vi "Address Lookup Table Initialize.vi"(8 "error in (no error)":errorcluster) -> (0 "error out":errorcluster {"code" min=0 max=0}, 3 "reference out 2":T1)   [LabVIEW 2013, in "J1939 Addon Engine.lvlib"]
uses:
  J1939 Addon Engine.lvlib
  Shared/J1939 Multi Packet Frame/Types/Address Table Reference.ctl
  Shared/J1939 Multi Packet Frame/Types/Address Lookup Table Action.ctl
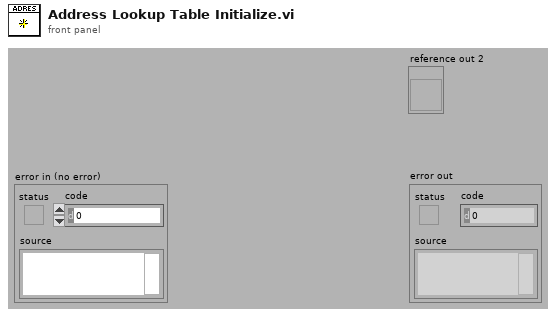
[diagram p1: front panel]
types:
  T1 = typedef "J1939 Addon Engine.lvlib/Address Table Reference.ctl" = refnum<vi>
  T2 = typedef "J1939 Addon Engine.lvlib/Address Lookup Table Action.ctl" = enum16{"Initialize", "Add", "Get", "Remove", "Get All"}
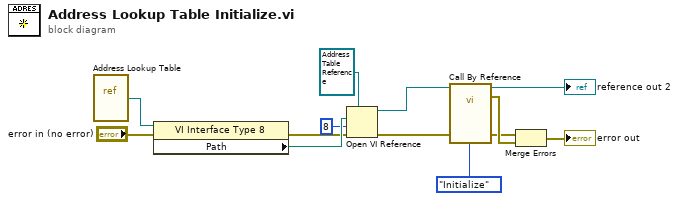
[diagram p0: block diagram]
diagram:
  n1 = vi-ref "Address Lookup Table.vi"() -> (w13:refnum<vi>)
  n2 = property class="VI Interface Type 8"(reference=w13, error in="error in (no error)") -> (error out=w10:errorcluster, "Path"=w12:path)  [unwired: 1 out]
  n3 = Open VI Reference(type specifier VI Refnum (for type only)=T1 refnum ("reference out 2"), vi path=w12, options=8, error in (no error)=w10) -> (vi reference=w9:T1, error out=w5:errorcluster)  [unwired: 2 in]
  n4 = call-by-ref "?"(reference=w9, "Action"=Address_Lookup_Table_Action."Initialize", "error in (no error)"=w5) -> (reference out=→"reference out 2":T1, error out=w8:errorcluster, 0:"error out"=w4:errorcluster)  [unwired: 7 in, 3 out]
  n5 = Merge Errors(w4, w8) -> (→"error out":errorcluster)
